vi "System Required Helper.vi"(8 "System Required Argument":T2, 11 "Module Data":T3) -> (0 "System Required (Reply Payload)":T1, 1 "Message":string, 3 "Module Data out":T3)   [LabVIEW 2024, in "DQMH Power Requests.lvlib"]
doc: "<b>Note:</b> This VI was modified by the <b>Validate DQMH Module</b> tool to turn off automatic error handling.\n\n<b>Note:</b> This VI was modified by the <b>Validate DQMH Module</b> tool to be shared clone reentrant."
uses:
  DQMH Power Requests.lvlib
  Module Data--cluster.ctl
  System Required Argument--cluster.ctl
  System Required (Reply Payload)--cluster.ctl
  Power-Requests/Power Availabilty Requests/Type Defs/Power Availiability Requests Functions.ctl
  Power-Requests/Power Availabilty Requests/Type Defs/Power Request Type.ctl
  <vilib>/Utility/error.llb/Error Cluster From Error Code.vi
  <vilib>/ErrorRing/Error Ring.xnode
  Power-Requests/Power Requests.lvlib
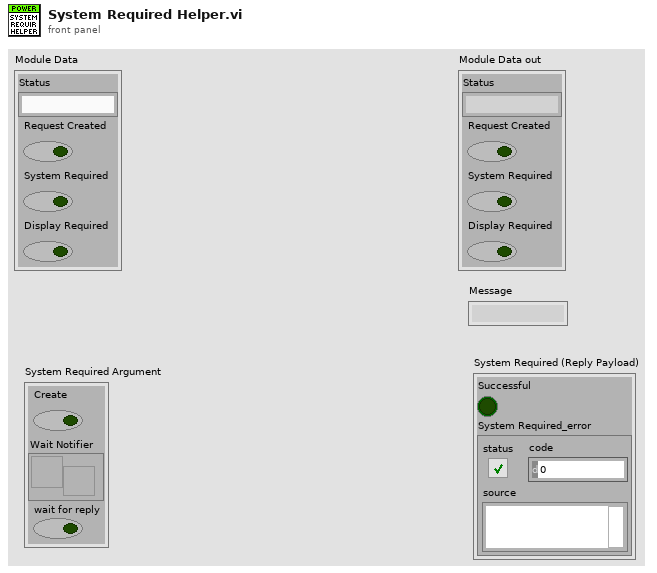
[diagram p1: front panel]
types:
  T1 = typedef "DQMH Power Requests.lvlib/System Required (Reply Payload)--cluster.ctl" = cluster{"Successful":bool, "System Required_error":errorcluster}
  T2 = typedef "DQMH Power Requests.lvlib/System Required Argument--cluster.ctl" = cluster{"Create":bool, "Wait Notifier":refnum<notifier>, "wait for reply":bool}
  T3 = typedef "DQMH Power Requests.lvlib/Module Data--cluster.ctl" = cluster{"Status":string, "Request Created":bool, "System Required":bool, "Display Required":bool}
  T4 = typedef "Power Requests.lvlib/Power Request Type.ctl" = enum32{"Power Request Display Required", "Power Request System Required", "Power Request Away Mode Required", "Power Request Execution Required"}
  T5 = typedef "Power Requests.lvlib/Power Availiability Requests Functions.ctl" = enum32{"Power Create Request", "Power Set Request", "Power Clear Request", "Close Handle"}
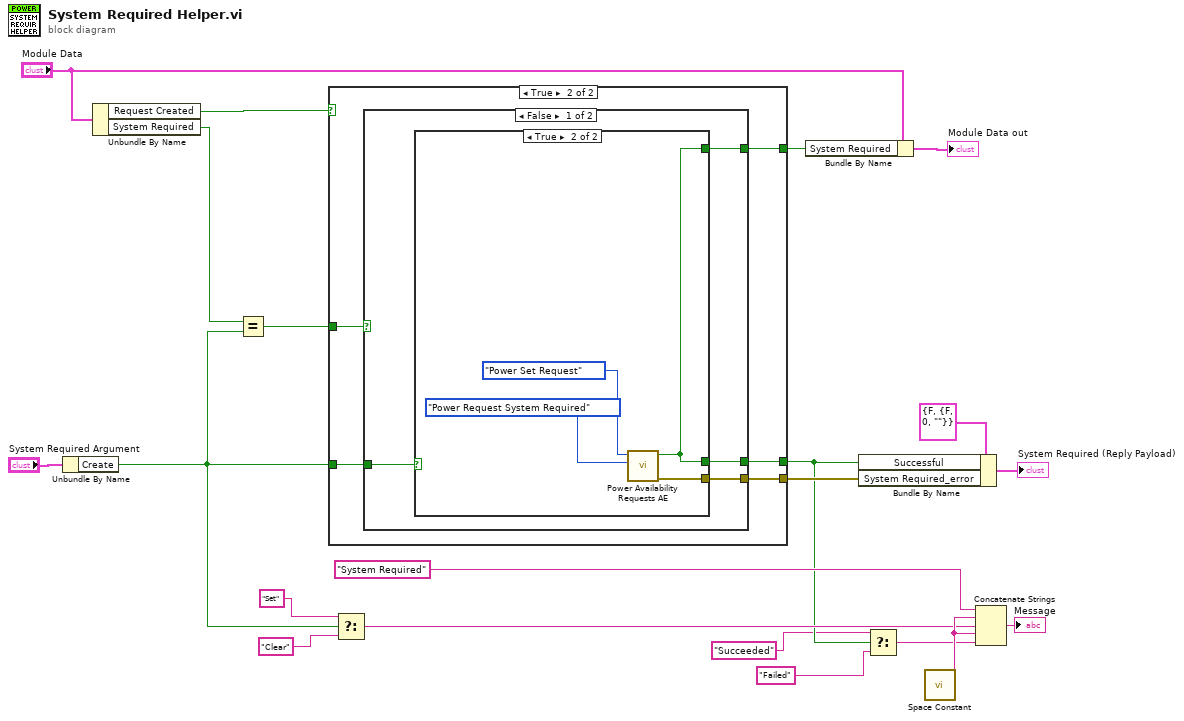
[diagram p0: block diagram]
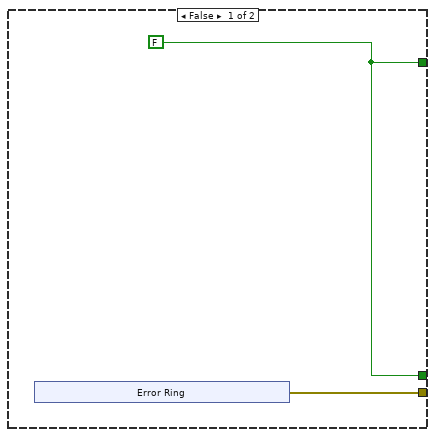
[diagram p2: hidden frame]
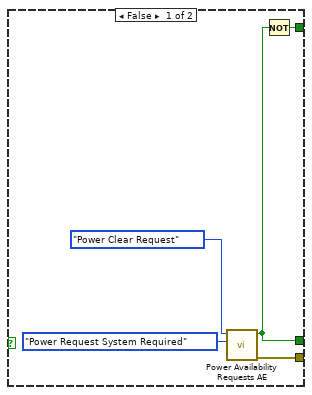
[diagram p3: hidden frame]
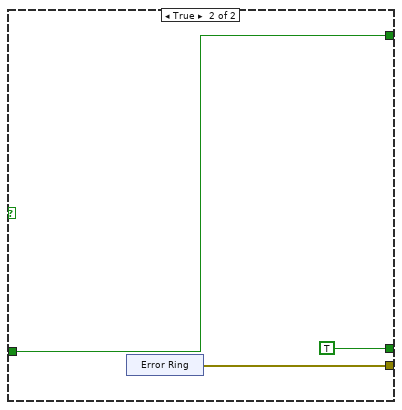
[diagram p4: hidden frame]
diagram:
  n1 = Unbundle By Name("System Required Argument") -> ("Create"=w8:bool)
  n2 = Unbundle By Name("Module Data") -> ("Request Created"=w16:bool, "System Required"=w12:bool)
  n3 = Equal?(x=w12, y=w8) -> (x = y?=w13:bool)
  n4 = case shown="True" w16 {
    tunnel: [w23 w31] -> w15
    tunnel: [w23 w29] -> w3
    tunnel: [w22 w28] -> w14
    tunnel: w13 -> [_ w32]
    tunnel: w8 -> [_ w30]
    frame False {
      w23 = FALSE
      n5 = xnode "Error Ring"() -> ("error out"=w22:errorcluster)
    }
    frame True {
      n6 = case shown="False" w32 {
        tunnel: [w33 w48] -> w31
        tunnel: w30 -> [w36 w48]
        tunnel: [w34 TRUE] -> w29
        tunnel: [w35 w46] -> w28
        frame False {
          n7 = case shown="True" w36 {
            tunnel: [w41 w45] -> w35
            tunnel: [w38 w44] -> w34
            tunnel: [w37 w44] -> w33
            frame False {
              n8 = call "Power Availability Requests AE.vi"("Power Request Type"=Power_Request_Type."Power Request System Required", "Power Availability Requests Functions"=Power_Availiability_Requests_Functions."Power Clear Request") -> ("error out"=w41:errorcluster, "Success?"=w38:bool)  [unwired: 8 in]
              n9 = Not(x=w38) -> (.not. x?=w37:bool)
            }
            frame True {
              n10 = call "Power Availability Requests AE.vi"("Power Request Type"=Power_Request_Type."Power Request System Required", "Power Availability Requests Functions"=Power_Availiability_Requests_Functions."Power Set Request") -> ("error out"=w45:errorcluster, "Success?"=w44:bool)  [unwired: 8 in]
            }
          }
        }
        frame True {
          n11 = xnode "Error Ring"() -> ("error out"=w46:errorcluster)
        }
      }
    }
  }
  n12 = Select(t="Set", s=w8, f="Clear") -> (s? t:f=w5:string)
  n13 = Bundle By Name(cluster="Module Data", "System Required"=w15) -> (→"Module Data out":T3)
  n14 = Bundle By Name(cluster=T1 {"Successful"=FALSE, "System Required_error"={"status"=FALSE, "code"=0, "source"=""}} ("System Required (Reply Payload)"), "Successful"=w3, "System Required_error"=w14) -> (→"System Required (Reply Payload)":T1)
  n15 = Select(t="Succeeded", s=w3, f="Failed") -> (s? t:f=w4:string)
  n16 = call <vilib>:"Space Constant.vi"() -> ("String"=w9:string)
  n17 = Concatenate Strings("System Required", w9, w5, w9, w4) -> (→"Message":string)
